vi "SaveWaveformData.vi"(5 "Registry":T15, 6 "data event data":T1, 7 "error in (no error)":errorcluster, 9 "waveform data":waveform(sgl)[](array[waveform]), 10 "data event":T9) -> (0 "error out":errorcluster, 3 "data event data out":T1)   [LabVIEW 2017, in "McsaDataEventCreator.lvlib"]
uses:
  <vilib>/addons/InsightCM/Devices/Shared/Mcsa/McsaDataEventCreator/McsaDataEventCreator.lvlib
  <vilib>/addons/InsightCM/Devices/Shared/Mcsa/McsaDataEventCreator/controls/DataGroupRegistry.ctl
  <vilib>/addons/InsightCM/Devices/Shared/Mcsa/McsaDataEventCreator/controls/Registry_DataSet.ctl
  <vilib>/addons/InsightCM/Devices/Shared/Mcsa/McsaDataEventCreator/controls/DataSetType.ctl
  <vilib>/addons/InsightCM/Devices/Shared/Common/DataEventCreator/controls/Registry_Trend.ctl
  <vilib>/addons/InsightCM/Devices/Shared/Mcsa/McsaDataEventCreator/controls/DataEventConfig.ctl
  <vilib>/addons/InsightCM/Devices/Shared/Mcsa/McsaDataEventCreator/controls/AcqParams.ctl
  <vilib>/addons/InsightCM/Devices/Shared/Common/DataAccumulator/controls/AccumulationSettings.ctl
  <vilib>/addons/InsightCM/Devices/Shared/Common/DataAccumulator/controls/accumulationType.ctl
  <vilib>/addons/InsightCM/Devices/Shared/Common/DVRBuffer/controls/BufferLocation.ctl
  <vilib>/addons/PointValueMap/controls/PointMap.ctl
  <vilib>/addons/InsightCM/Devices/Shared/Common/DataEvent/controls/Event.ctl
  <vilib>/addons/InsightCM/MessageBus/Base/controls/DataEvent.ctl
  <vilib>/addons/InsightCM/MessageBus/Base/controls/KeyValuePair.ctl
  <vilib>/addons/InsightCM/Devices/Shared/Common/DataEvent/controls/DataSet.ctl
  <vilib>/addons/InsightCM/MessageBus/Base/controls/DataSetMetadata.ctl
  <vilib>/addons/InsightCM/MessageBus/Base/controls/TrendPoint.ctl
  <vilib>/addons/InsightCM/MessageBus/Base/controls/TrendAlarmUpdate.ctl
  <vilib>/addons/InsightCM/MessageBus/Base/controls/TrendAlarmTransition.ctl
  <vilib>/addons/PointValueMap/PointValueMap.lvlib
  <vilib>/addons/InsightCM/Devices/Shared/Common/DataEventCreator/DataEventCreator.lvlib
  <vilib>/addons/InsightCM/Devices/Shared/Common/DataAccumulator/DataAccumulator.lvlib
  <vilib>/addons/InsightCM/Devices/Shared/Common/DVRBuffer/DVRBuffer.lvlib
  <vilib>/addons/InsightCM/Devices/Shared/Common/DataEvent/DataEvent.lvlib
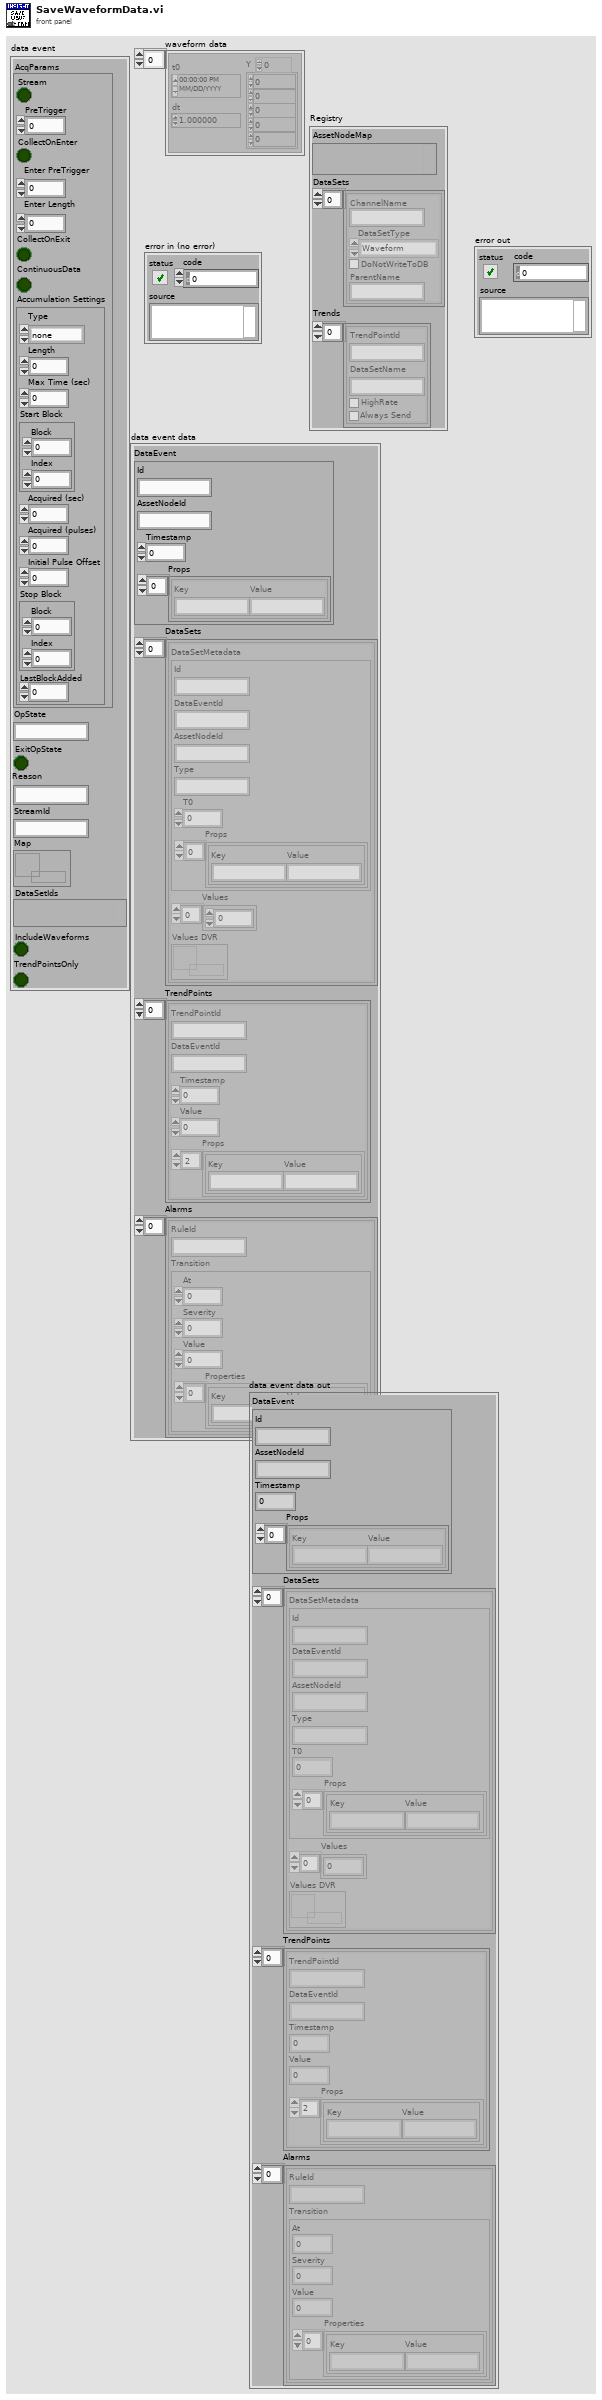
[diagram p1: front panel]
types:
  T1 = typedef "DataEvent.lvlib/Event.ctl" = cluster{"DataEvent":T2, "DataSets":T4[], "TrendPoints":T6[], "Alarms":T7[]}
  T2 = typedef "DataEvent.ctl" = cluster{"Id":string, "AssetNodeId":string, "Timestamp":i64, "Props":T3[]}
  T3 = typedef "KeyValuePair.ctl" = cluster{"Key":string, "Value":string}
  T4 = typedef "DataEvent.lvlib/DataSet.ctl" = cluster{"DataSetMetadata":T5, "Values":sgl[], "Values DVR":refnum<data-value>}
  T5 = typedef "DataSetMetadata.ctl" = cluster{"Id":string, "DataEventId":string, "AssetNodeId":string, "Type":string, "T0":i64, "Props":T3[]}
  T6 = typedef "TrendPoint.ctl" = cluster{"TrendPointId":string, "DataEventId":string, "Timestamp":i64, "Value":dbl, "Props":T3[]}
  T7 = typedef "TrendAlarmUpdate.ctl" = cluster{"RuleId":string, "Transition":T8}
  T8 = typedef "TrendAlarmTransition.ctl" = cluster{"At":i64, "Severity":i32, "Value":dbl, "Properties":T3[]}
  T9 = typedef "McsaDataEventCreator.lvlib/DataEventConfig.ctl" = cluster{"AcqParams":T10, "OpState":string, "ExitOpState":bool, "Reason":string, "StreamId":string, "Map":T14, "DataSetIds":variant, "IncludeWaveforms":bool, "TrendPointsOnly":bool}
  T10 = typedef "McsaDataEventCreator.lvlib/AcqParams.ctl" = cluster{"Stream":bool, "PreTrigger":i32, "CollectOnEnter":bool, "Enter PreTrigger":i32, "Enter Length":dbl, "CollectOnExit":bool, "ContinuousData":bool, "Accumulation Settings":T11}
  T11 = typedef "DataAccumulator.lvlib/AccumulationSettings.ctl" = cluster{"Type":T12, "Length":dbl, "Max Time (sec)":dbl, "Start Block":T13, "Acquired (sec)":dbl, "Acquired (pulses)":i32, "Initial Pulse Offset":dbl, "Stop Block":T13, "LastBlockAdded":u32}
  T12 = typedef "DataAccumulator.lvlib/accumulationType.ctl" = enum16{"none", "seconds", "revolutions"}
  T13 = typedef "DVRBuffer.lvlib/BufferLocation.ctl" = cluster{"Block":u32, "Index":i32}
  T14 = typedef "PointValueMap.lvlib/PointMap.ctl" = refnum<data-value>
  T15 = typedef "McsaDataEventCreator.lvlib/DataGroupRegistry.ctl" = cluster{"AssetNodeMap":variant, "DataSets":T16[], "Trends":T18[]}
  T16 = typedef "McsaDataEventCreator.lvlib/Registry_DataSet.ctl" = cluster{"ChannelName":string, "DataSetType":T17, "DoNotWriteToDB":bool, "ParentName":string}
  T17 = typedef "McsaDataEventCreator.lvlib/DataSetType.ctl" = enum16{"Waveform", "MCSAFFT", "TorqueWFM"}
  T18 = typedef "DataEventCreator.lvlib/Registry_Trend.ctl" = cluster{"TrendPointId":string, "DataSetName":string, "HighRate":bool, "Always Send":bool}
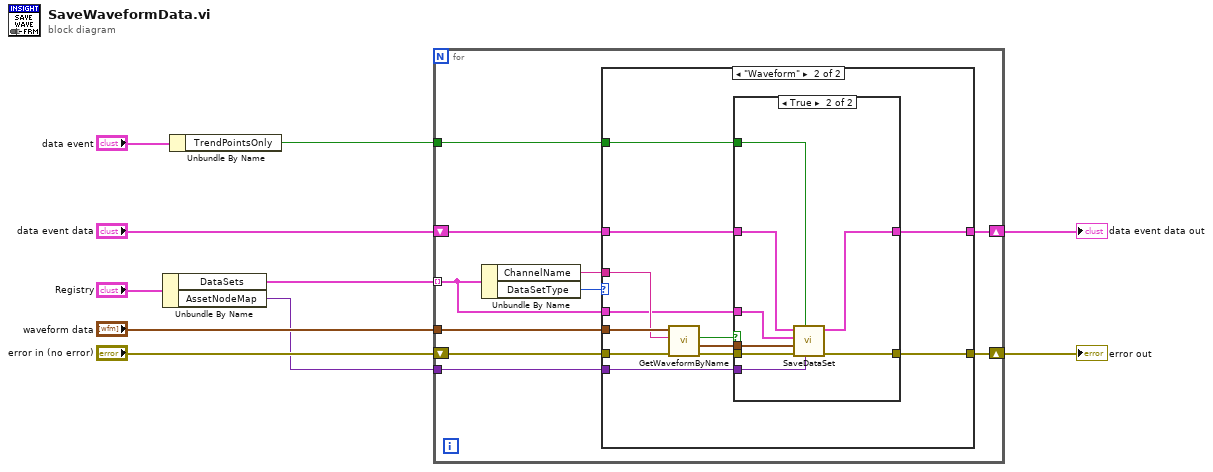
[diagram p0: block diagram]
diagram:
  n1 = Unbundle By Name("Registry") -> ("DataSets"=w7:T16[], "AssetNodeMap"=w5:variant)
  n2 = Unbundle By Name("data event") -> ("TrendPointsOnly"=w4:bool)
  n3 = for {
    tunnel: "waveform data" -> [w19]
    tunnel: w7 -> [w14] mode=indexing
    shift-right: [w18] -> w6
    shift-left: "error in (no error)" -> [w20]
    tunnel: w5 -> [w15]
    tunnel: w4 -> [w13]
    shift-right: [w11] -> w1
    shift-left: "data event data" -> [w12]
    n4 = Unbundle By Name(w14) -> ("ChannelName"=w17:string, "DataSetType"=w16:T17)
    n5 = case shown="\"Waveform\"" w16 {
      tunnel: w20 -> [w21 w34]
      tunnel: w19 -> [_ w33]
      tunnel: [w21 w32] -> w18
      tunnel: w17 -> [_ w31]
      tunnel: w12 -> [w22 w30]
      tunnel: w15 -> [_ w29]
      tunnel: w14 -> [_ w28]
      tunnel: [w22 w27] -> w11
      tunnel: w13 -> [_ w23]
      frame Default {
      }
      frame "Waveform" {
        n6 = call <vilib>:"GetWaveformByName.vi"("error in (no error)"=w34, "Channel Name"=w31, "Acq Waveforms"=w33) -> ("error out"=w26:errorcluster, "Waveform"=w25:waveform(sgl), "Found?"=w24:bool)  [unwired: 5 in, 1 out]
        n7 = case shown="True" w24 {
          tunnel: w26 -> [w36 w44]
          tunnel: w25 -> [_ w43]
          tunnel: [w36 w38] -> w32
          tunnel: w30 -> [w35 w42]
          tunnel: w29 -> [_ w41]
          tunnel: w28 -> [_ w40]
          tunnel: [w35 w39] -> w27
          tunnel: w23 -> [_ w37]
          frame False {
          }
          frame True {
            n8 = call <vilib>:"SaveDataSet.vi"("AssetNodeMap"=w41, "do not write to database"=w37, "error in (no error)"=w44, "Waveform"=w43, "DataSetRegistry"=w40, "event in"=w42) -> ("error out"=w38:errorcluster, "event out"=w39:T1)  [unwired: 4 in]
          }
        }
      }
    }
  }
  "error out" <- w6
  "data event data out" <- w1
